vi "iVIO Test.vi"(6 "script name":string="LPtoActive", 8 "error in (no error)":errorcluster, 9 "Publishable IDs":string[](array[string])=["IDD_LowPower", "IDD_DVC_Cmin", "IDD_DVC_Cmax"], 10 "Pins":string[](array[string])=["VDD"], 11 "Semiconductor Module Context":T1) -> (0 "error out":errorcluster)   [LabVIEW 2013]
uses:
  <vilib>/NI_TestStand_SemiconductorModule/NI_TestStand_Semiconductor_Module.lvlibp/PinMap/General/SemiconductorModuleContext.ctl
  <instrlib>/niHSDIO/niHSDIO.llb/niHSDIO_ctl Trigger Script - trigID Values (Ring).ctl
  <vilib>/NI_TestStand_SemiconductorModule/NI_TestStand_Semiconductor_Module.lvlibp/PinMap/DC Power/PinsToNIDCPowerSessions.vi
  <vilib>/NI_TestStand_SemiconductorModule/NI_TestStand_Semiconductor_Module.lvlibp/PinMap/General/Publish/PublishDataDouble2D.vi
  <vilib>/NI_TestStand_SemiconductorModule/NI_TestStand_Semiconductor_Module.lvlibp
panel:
  out "current measurements":dbl[][](array[numeric])
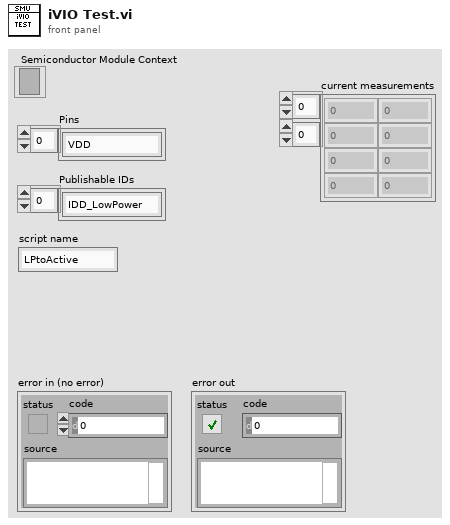
[diagram p1: front panel]
types:
  T1 = typedef "NI_TestStand_Semiconductor_Module.lvlibp/SemiconductorModuleContext.ctl" = refnum<k7>
  T2 = typedef "niHSDIO_ctl Trigger Script - trigID Values (Ring).ctl" = string
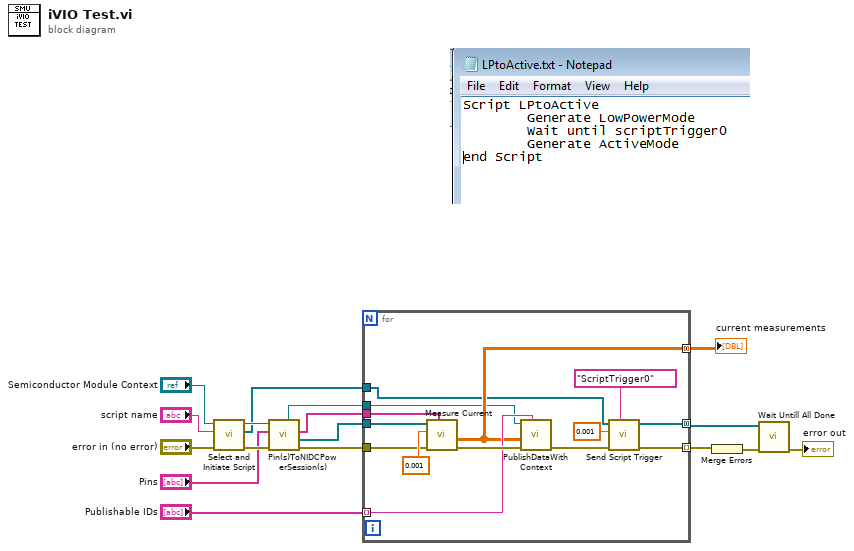
[diagram p0: block diagram]
diagram:
  n1 = call "Select and Initiate Script.vi"("error in (no error)"="error in (no error)", "script name"="script name", "Semiconductor Module Context"="Semiconductor Module Context") -> ("error out"=w11:errorcluster, "HSDIO GEN Sessions Out"=w4:refnum<k15>[], "Semiconductor Module Context Out"=w10:T1)  [unwired: 6 in]
  n2 = call-poly <vilib>:"Pin(s)ToNIDCPowerSession(s).vi"("error in (no error)"=w11, "Pins"="Pins", "Semiconductor Module Context"=w10) -> ("error out"=w8:errorcluster, "Instrument Sessions"=w7:refnum<k15>[], "Channel Lists"=w6:string[], "Pin Query Context"=w5:refnum<class "MultiplePinMultipleSessionQueryContext.lvclass">)  [unwired: 4 in, 1 out]
  n3 = for {
    tunnel: "Publishable IDs" -> [w30] mode=indexing
    tunnel: [w28] -> w13 mode=concatenating
    tunnel: w8 -> [w25]
    tunnel: w7 -> [w24]
    tunnel: w6 -> [w23]
    tunnel: w5 -> [w22]
    tunnel: w4 -> [w20]
    tunnel: [w19] -> w3 mode=indexing
    tunnel: [w18] -> w1 mode=concatenating
    n4 = call "Measure Current.vi"("Channel Lists"=w23, "error in (no error)"=w25, "Delay Time (s)"=0.001, "DCPower Sessions In"=w24) -> ("error out"=w31:errorcluster, "current measurements"=w28:dbl[][])  [unwired: 5 in, 1 out]
    n5 = call-poly <vilib>:"PublishDataWithContext.vi"("Published Data Id"=w30, "error in (no error)"=w31, "Data In"=w28, "Pin Query Context"=w22) -> ("error out"=w21:errorcluster)  [unwired: 6 in, 1 out]
    n6 = call "Send Script Trigger.vi"("trigger id (script trigger 0)"=T2 "ScriptTrigger0", "error in (no error)"=w21, "Delay Time (s)"=0.001, "HSDIO Sessions In"=w20) -> ("error out"=w19:errorcluster, "HSDIO Sessions Out"=w18:refnum<k15>[])  [unwired: 6 in]
  }
  "current measurements" <- w13
  n7 = Merge Errors(w3) -> (w2:errorcluster)
  n8 = call "Wait Untill All Done.vi"("error in (no error)"=w2, "HSDIO Sessions In"=w1) -> ("error out"=→"error out":errorcluster)  [unwired: 8 in, 1 out]
